vi "Equal.vi"(1 "Input2":dbl format="%.2f", 2 "Input1":dbl format="%.2f") -> (0 "Equal?":bool)   [LabVIEW 2020]
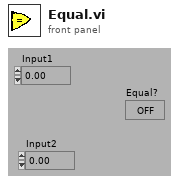
[diagram p1: front panel]
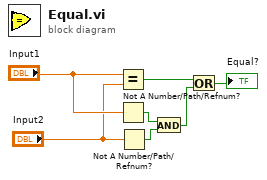
[diagram p0: block diagram]
diagram:
  n1 = Equal?(x="Input1", y="Input2") -> (x = y?=w6:bool)
  n2 = Not A Number/Path/Refnum?(number/path/refnum="Input1") -> (NaN/Path/Refnum?=w4:bool)
  n3 = Not A Number/Path/Refnum?(number/path/refnum="Input2") -> (NaN/Path/Refnum?=w3:bool)
  n4 = And(x=w4, y=w3) -> (x .and. y?=w5:bool)
  n5 = Or(x=w6, y=w5) -> (x .or. y?=→"Equal?":bool)
